vi "Continuous Waveform Convolution for N Chan.vi"(6 "delay output with half kernel length":bool, 7 "reset":bool, 8 "error in (no error)":errorcluster, 9 "algorithm":enum32{"direct", "frequency domain"}(ring)=enum."frequency domain", 10 "kernels":dbl[][](array[numeric]), 11 "signals in":waveform(dbl)[](array[waveform])) -> (0 "error out":errorcluster, 3 "signals out":waveform(dbl)[](array[waveform]))   [LabVIEW 2020, in "NI_MAPro.lvlib"]
doc: "Convolves single or multiple waveforms and one or more kernels with state, allowing subsequent calls to be processed in a continuous manner. If you are convolving multiple waveforms, the VI maintains separate convolution states for each waveform."
uses:
  NI_MAPro.lvlib
  NI_MABase.lvlib
panel:
  # "Continuous Convolutions with 2D Kernel Array"
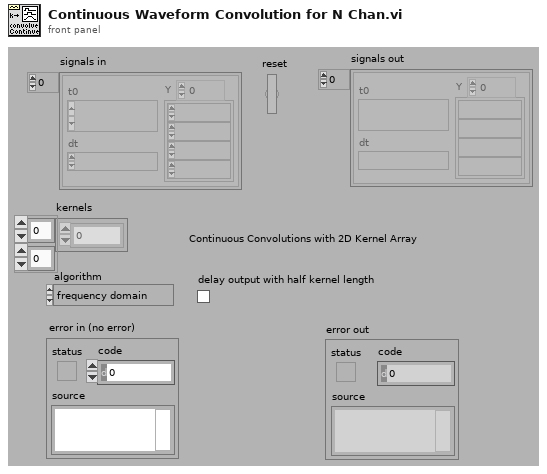
[diagram p1: front panel]
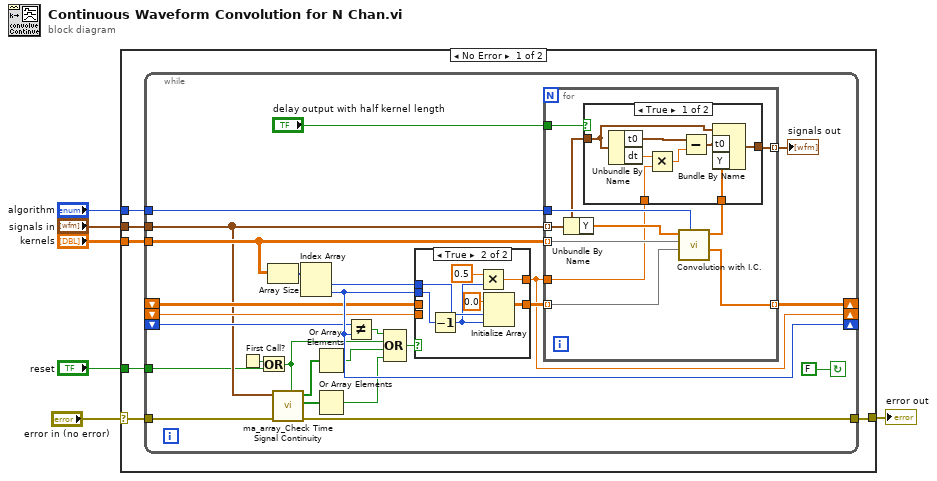
[diagram p0: block diagram]
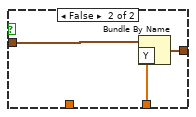
[diagram p3: hidden frame]
diagram:
  n1 = case shown="No Error" "error in (no error)" {
    selector: "error in (no error)" -> [w8 w69]
    tunnel: [w7 w69] -> w5
    tunnel: "algorithm" -> [w12 _]
    tunnel: "signals in" -> [w11 _]
    tunnel: "kernels" -> [w10 _]
    tunnel: "reset" -> [w9 _]
    frame No Error {
      n2 = while {
        shift-right: [w36] -> _
        shift-left: _ -> [w30]
        shift-right: [w38] -> _
        shift-left: _ -> [w25]
        shift-right: [w27] -> _
        shift-left: _ -> [w26]
        tunnel: w12 -> [w24]
        tunnel: w11 -> [w22]
        tunnel: w10 -> [w23]
        tunnel: w9 -> [w21]
        tunnel: w8 -> [w14]
        tunnel: [w13] -> w7
        stop <- FALSE continue-if-true
        n3 = First Call?() -> (First Call?: T/F=w20:bool)
        n4 = Or(x=w20, y=w21) -> (x .or. y?=w19:bool)
        n5 = Array Size(array=w23) -> (size(s)=w33:i32[])
        n6 = call "ma_array_Check Time Signal Continuity.vi"("Ignore input time stamp"=w19, "error in (no error)"=w14, "waveforms"=w22) -> ("error out"=w13:errorcluster, "dt changed"=w17:bool[], "t0 changed"=w18:bool[])  [unwired: 5 in, 1 out]
        n7 = Index Array(array=w33) -> (element #1=w28:i32, element #2=w38:i32)  [unwired: 2 in]
        n8 = Or Array Elements(Boolean array=w18) -> (logical OR=w16:bool)
        n9 = Or Array Elements(Boolean array=w17) -> (logical OR=w15:bool)
        n10 = Not Equal?(x=w25, y=w38) -> (x != y?=w32:bool)
        n11 = Compound Arithmetic op=OR(w32, w19, w16, w15) -> (w29:bool)
        n12 = case shown="True" w29 {
          tunnel: [w40 w47] -> w31
          tunnel: w30 -> [w40 _]
          tunnel: w28 -> [_ w46]
          tunnel: w38 -> [_ w45]
          tunnel: [w39 w41] -> w27
          tunnel: w26 -> [w39 _]
          frame False {
          }
          frame True {
            n13 = Decrement(x=w45) -> (x-1=w43:i32)
            n14 = Multiply(x=0.5, y=w43) -> (x*y=w41:dbl)
            n15 = Initialize Array(0.0 ("element"), w46, w43) -> (w47:dbl[][])
          }
        }
        n16 = for {
          tunnel: w31 -> [w49] mode=indexing
          tunnel: [w57] -> w36 mode=indexing
          tunnel: w24 -> [w56]
          tunnel: w23 -> [w55] mode=indexing
          tunnel: "delay output with half kernel length" -> [w52]
          tunnel: [w51] -> w34 mode=indexing
          tunnel: w22 -> [w50] mode=indexing
          tunnel: w27 -> [w48]
          n17 = Unbundle By Name(w50) -> ("Y"=w54:dbl[])
          n18 = call "Convolution with I.C..vi"("algorithm"=w56, "Initial conditions"=w49, "Kernel"=w55, "Array in"=w54) -> ("final conditions"=w57:dbl[], "Array out"=w53:dbl[])  [unwired: 2 in, 1 out]
          n19 = case shown="True" w52 {
            tunnel: [w65 w68] -> w51
            tunnel: w53 -> [w64 w67]
            tunnel: w50 -> [w63 w66]
            tunnel: w48 -> [w59 _]
            frame True {
              n20 = Unbundle By Name(w63) -> ("t0"=w61:timestamp, "dt"=w60:dbl)
              n21 = Multiply(x=w60, y=w59) -> (x*y=w58:dbl)
              n22 = Subtract(x=w61, y=w58) -> (x-y=w62:timestamp)
              n23 = Bundle By Name(cluster=w63, "t0"=w62, "Y"=w64) -> (w65:waveform(dbl))
            }
            frame False {
              n24 = Bundle By Name(cluster=w66, "Y"=w67) -> (w68:waveform(dbl))
            }
          }
        }
        "signals out" <- w34
      }
    }
    frame Error {
    }
  }
  "error out" <- w5
